vi "Frameremap.vi"(10 "Size (m)":cluster{"Width":sgl, "Height":sgl} {"Height" format="%.2p"; "Width" format="%.2p"}, 11 "Origin (m)":cluster{"Xc":sgl, "Yc":sgl} {"Yc" format="%.2p"; "Xc" format="%.2p"}) -> (3 "Remapped Frame Properties":T1)   [LabVIEW 2019]
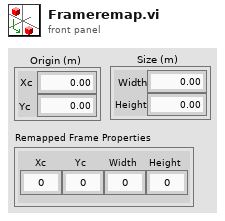
[diagram p1: front panel]
types:
  T1 = cluster{"Xc":dbl, "Yc":dbl, "Width":dbl, "Height":dbl}
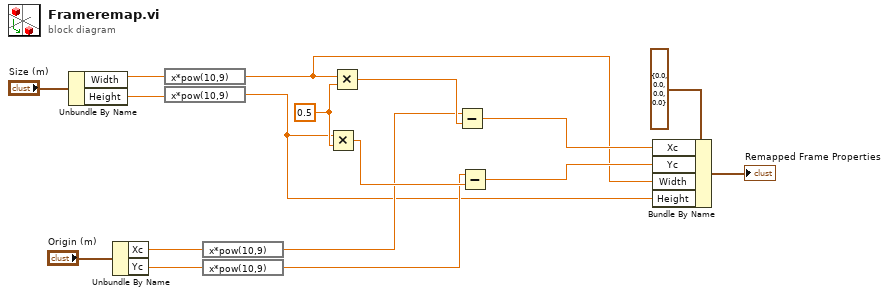
[diagram p0: block diagram]
diagram:
  w17 = 0.5 ("y")
  n1 = Unbundle By Name("Size (m)") -> ("Width"=w12:sgl, "Height"=w11:sgl)
  n2 = Unbundle By Name("Origin (m)") -> ("Xc"=w10:sgl, "Yc"=w7:sgl)
  n3 = expression code="x*pow(10,9)"(w12) -> (w2:sgl)
  n4 = expression code="x*pow(10,9)"(w11) -> (w1:sgl)
  n5 = expression code="x*pow(10,9)"(w10) -> (w9:sgl)
  n6 = expression code="x*pow(10,9)"(w7) -> (w8:sgl)
  n7 = Multiply(x=w1, y=w17) -> (x*y=w15:dbl)
  n8 = Multiply(x=w2, y=w17) -> (x*y=w16:dbl)
  n9 = Subtract(x=w9, y=w16) -> (x-y=w3:dbl)
  n10 = Subtract(x=w8, y=w15) -> (x-y=w4:dbl)
  n11 = Bundle By Name(cluster=T1 {"Xc"=0.0, "Yc"=0.0, "Width"=0.0, "Height"=0.0} ("Remapped Frame Properties"), "Xc"=w3, "Yc"=w4, "Width"=w2, "Height"=w1) -> (→"Remapped Frame Properties":T1)
